vi "Enqueue Return Value.vi"(8 "error in (no error)":errorcluster, 10 "This VI":refnum<vi>, 11 "Mock In":refnum<class "Responsive Mock.lvclass">) -> (0 "error out":errorcluster, 3 "Mock Out":refnum<class "Responsive Mock.lvclass">)   [LabVIEW 2020, in "Responsive Mock.lvclass"]
uses:
  Responsive Mock.lvclass
  Responsive Mock.lvclass/Responsive Mock.ctl
  Core/VI Call/VI Call.lvclass
  VI Server VI Call/VI Server VI Call.lvclass
  C:/git/astemes-lmock/source/Framework/VI Call/VI Call.lvclass
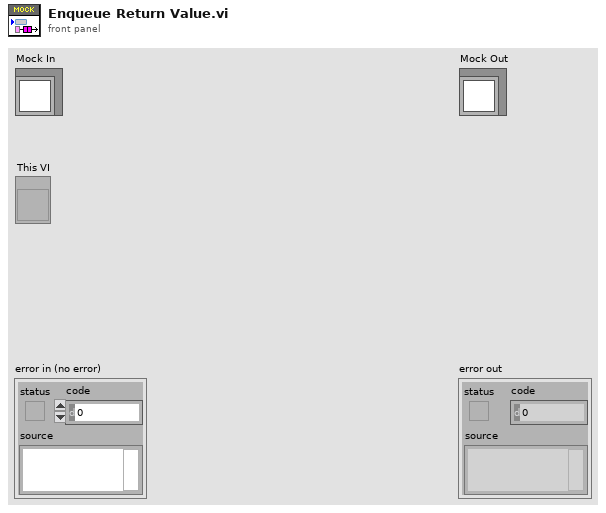
[diagram p1: front panel]
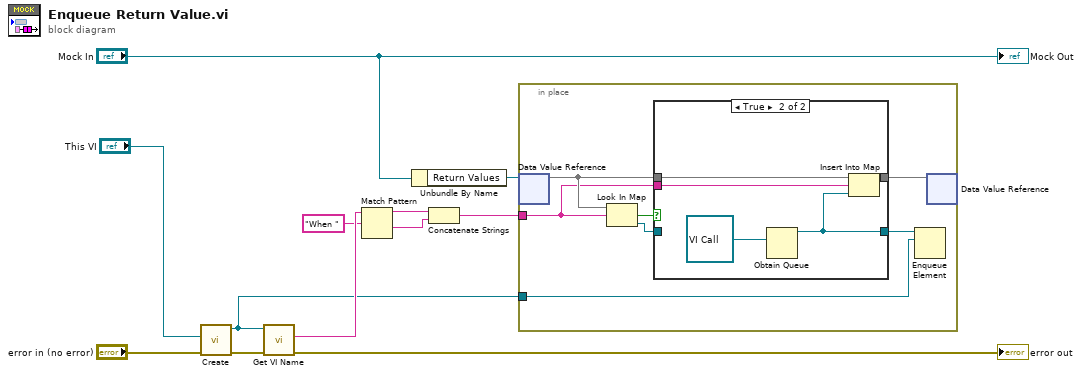
[diagram p0: block diagram]
diagram:
  n1 = call "Create.vi"("error in (no error)"="error in (no error)", "VI"="This VI") -> ("error out"=w10:errorcluster, "Call Out"=w1:refnum<class "VI Server VI Call.lvclass">)  [unwired: 8 in]
  n2 = call-dynamic "Get VI Name.vi"("error in (no error)"=w10, "VI Call in"=w1) -> ("error out"=→"error out":errorcluster, "VI Name"=w8:string)  [unwired: 8 in]
  n3 = Match Pattern(string=w8, regular expression="When ") -> (before substring=w6:string, after substring=w5:string)  [unwired: 1 in, 2 out]
  n4 = Unbundle By Name("Mock In") -> ("Return Values"=w3:refnum<data-value>)
  n5 = Concatenate Strings(w6, w5) -> (w2:string)
  n6 = in-place {
    in-place-border: w2 -> [w16]
    in-place-border: w1 -> [w13]
    n7 = in-place-dvr #1(w3) -> (w18:map{string, refnum<queue>})  [unwired: 1 out]
    n8 = Look In Map(map=w18, key=w16) -> (key not found?=w19:bool, value=w17:refnum<queue>)  [unwired: 1 in]
    n9 = case shown="True" w19 {
      tunnel: w18 -> [w21 w25]
      tunnel: w17 -> [w20 _]
      tunnel: w16 -> [_ w24]
      tunnel: [w21 w23] -> w15
      tunnel: [w20 w22] -> w14
      frame False {
      }
      frame True {
        n10 = Obtain Queue(element data type=refnum<class "VI Call.lvclass"> refnum ("Call Out")) -> (queue out=w22:refnum<queue>)  [unwired: 4 in, 2 out]
        n11 = Insert Into Map(map in=w25, key=w24, value=w22) -> (map out=w23:map{string, refnum<queue>})  [unwired: 2 out]
      }
    }
    n12 = Enqueue Element(queue=w14, element=w13) -> ()  [unwired: 2 in, 3 out]
    n13 = in-place-dvr #1(w15) -> ()  [unwired: 2 out]
  }
  "Mock Out" <- "Mock In"
